vi "Construct.vi"(6 "Logfile directory":path, 7 "Rollover (true)":bool=TRUE, 8 "Error in (no error)":errorcluster, 9 "Logfile name":string="%date%.log", 10 "LogFormatterInterface in":refnum<class "LogFormatterInterface.lvclass">) -> (0 "Error out":errorcluster, 3 "LogWriterStream out":refnum<class "LogWriterStream.lvclass">)   [LabVIEW 2011, in "LogWriterStream.lvclass"]
uses:
  LogWriterStream.lvclass
  Formatter/LogFormatterInterface/LogFormatterInterface.lvclass
  LogWriterStream.lvclass/LogWriterStream.ctl
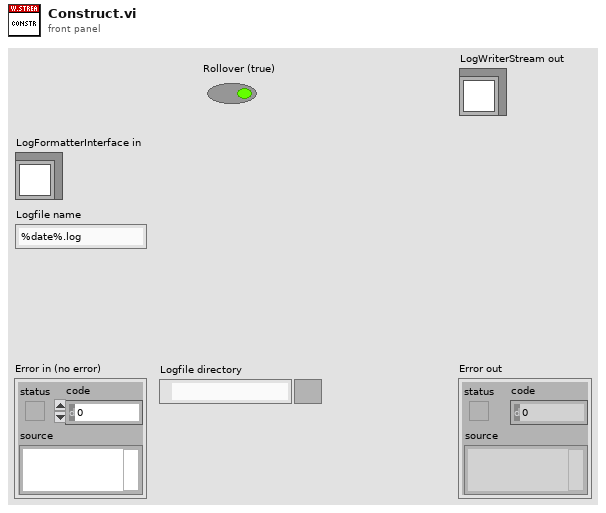
[diagram p1: front panel]
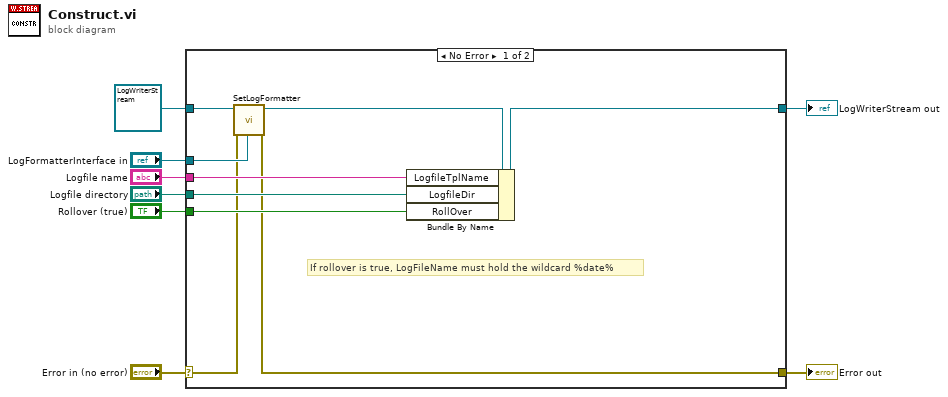
[diagram p0: block diagram]
diagram:
  n1 = case shown="No Error" "Error in (no error)" {
    selector: "Error in (no error)" -> [w10 w19]
    tunnel: [w9 w19] -> w7
    tunnel: [w14 w18] -> w6
    tunnel: refnum<class "LogWriterStream.lvclass"> refnum ("LogWriterStream in") -> [w13 w18]
    tunnel: "Logfile directory" -> [w16 _]
    tunnel: "Logfile name" -> [w17 _]
    tunnel: "Rollover (true)" -> [w15 _]
    tunnel: "LogFormatterInterface in" -> [w11 _]
    frame No Error {
      # "If rollover is true, LogFileName must hold the wildcard %date%"
      n2 = call-dynamic "SetLogFormatter.vi"("Error in (no error)"=w10, "LogFormatterInterface in"=w11, "LogWriterStream in"=w13) -> ("Error out"=w9:errorcluster, "LogWriterStream out"=w12:refnum<class "LogWriterStream.lvclass">)  [unwired: 7 in]
      n3 = Bundle By Name(cluster=w12, "LogfileTplName"=w17, "LogfileDir"=w16, "RollOver"=w15) -> (w14:refnum<class "LogWriterStream.lvclass">)
    }
    frame Error {
    }
  }
  "Error out" <- w7
  "LogWriterStream out" <- w6
